vi "HTTP DELETE.vi"(6 "request specific headers":T1[](array[typedef]), 7 "timeout (0 = Use Default)":i32, 8 "error in (no error)":errorcluster, 10 "Path":string, 11 "REST Client in":refnum<class "REST Client_JKI.lvclass">) -> (0 "error out":errorcluster, 1 "Response body":string, 2 "Response Headers":refnum<class "Response Headers.lvclass">, 3 "REST Client out":refnum<class "REST Client_JKI.lvclass">, 4 "Status String":string, 5 "Status Code":u16)   [LabVIEW 2018, in "REST Client.lvlib" / "REST Client_JKI.lvclass"]
doc: "Perform a HTTP DELETE request.\n\nThe VI provides multiple arguments for defining how to perform the HTTP request.\n\n<b>Path</b> specifies the path beneath the Base URL to be used for the HTTP request.\n\n<b>request specific headers</b> specifies an array of headers to be used with this particular HTTP request. The Default Headers specified upon creation of the JKI REST Client together with the request specific headers will all be used for the HTTP request."
uses:
  REST Client_JKI.lvclass
  Response Headers/Response Headers.lvclass
  REST Client/HTTP Header.ctl
  REST Client/HTTP Methods.ctl
  REST Client/REST Client.lvclass
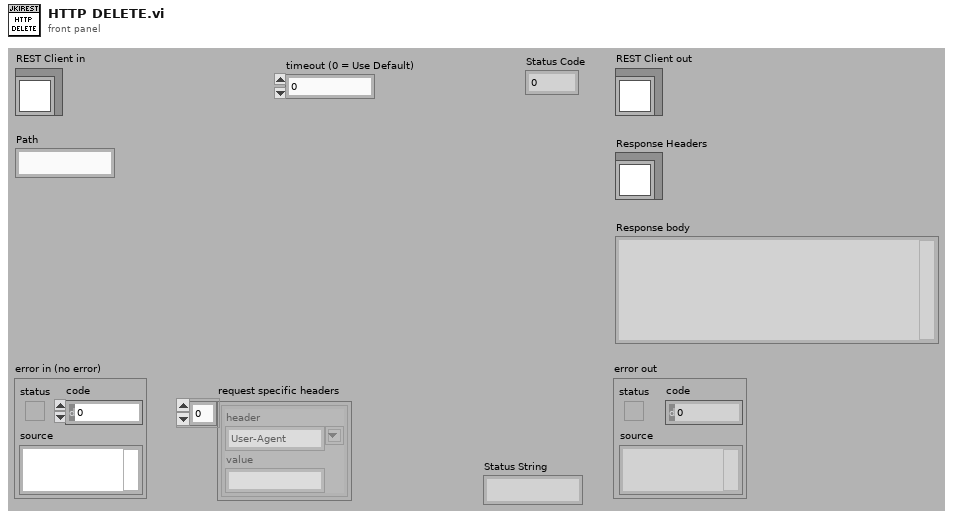
[diagram p1: front panel]
types:
  T1 = typedef "REST Client.lvlib/REST Client.lvclass/HTTP Header.ctl" = cluster{"header":string, "value":string}
  T2 = typedef "REST Client.lvlib/REST Client.lvclass/HTTP Methods.ctl" = enum16{"GET", "HEAD", "POST", "PUT", "DELETE"}
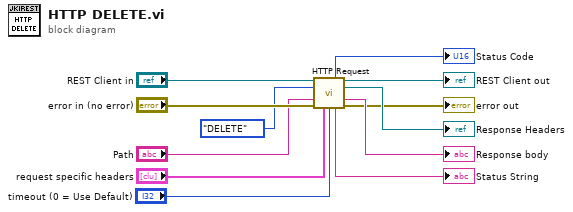
[diagram p0: block diagram]
diagram:
  n1 = call-dynamic "HTTP Request.vi"("REST Client in"="REST Client in", "Method"=HTTP_Methods."DELETE", "Path"="Path", "error in (no error)"="error in (no error)", "request specific headers"="request specific headers", "timeout (0 = Use Default)"="timeout (0 = Use Default)") -> ("Status Code"=→"Status Code":u16, "REST Client out"=→"REST Client out":refnum<class "REST Client_JKI.lvclass">, "Response Headers out"=→"Response Headers":refnum<class "Response Headers.lvclass">, "Response body"=→"Response body":string, "Status String"=→"Status String":string, "error out"=→"error out":errorcluster)  [unwired: 4 in]
